vi "Update Values.vi"(0 "Portfolio en entrée":refnum<class "Portfolio.lvclass"> caption="DNL_LabVIEW Object in", 5 "With Web Update ?":bool, 11 "error in (no error)":errorcluster caption="entrée d'erreur (pas d'erreur)") -> (4 "Portfolio en sortie":refnum<class "Portfolio.lvclass"> caption="DNL_LabVIEW Object out", 6 "Tableau":string[][](array[string]), 8 "Couleurs Change (%)":u32[](array[numeric]), 10 "Couleurs Obj":u32[](array[numeric]), 12 "Couleurs Stop (%)":u32[](array[numeric]), 13 "Calc Done ?":bool, 14 "Couleurs Dividende":u32[](array[numeric]), 15 "error out":errorcluster caption="sortie d'erreur")   [LabVIEW 2012, in "Portfolio.lvclass"]
uses:
  Portfolio.lvclass
  Stocks Manager/Stock Manager Action.ctl
  Portfolio.lvclass/Portfolio.ctl
  Stock/Stock.lvclass/Stock.ctl
  Stock/Stock.lvclass
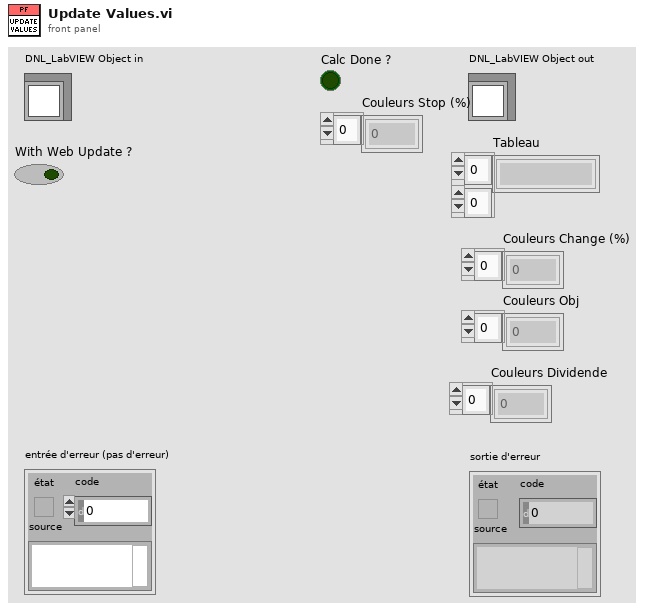
[diagram p1: front panel]
types:
  T1 = typedef "Stock Manager Action.ctl" = enum16{"Get_Stocks", "Load_Stocks", "Find_Stock_From_ISIN", "Find_Stock_From_Label", "Find_Stock_From_Symbol"}
  T2 = typedef "Stock.lvclass/Stock Parameters.ctl" = cluster{"Label":string, "Symbol":string, "Dividend":dbl, "Currency":T3, "ISIN":string, "Symbol_Suffix":string, "Last Price":dbl, "Dividend-Date":string, "Change (%)":dbl, "Objective":dbl, "Stop":dbl}
  T3 = typedef "Currencies.ctl" = enum16{"Euro", "Dollar", "Yen", "RIM", "CHF"}
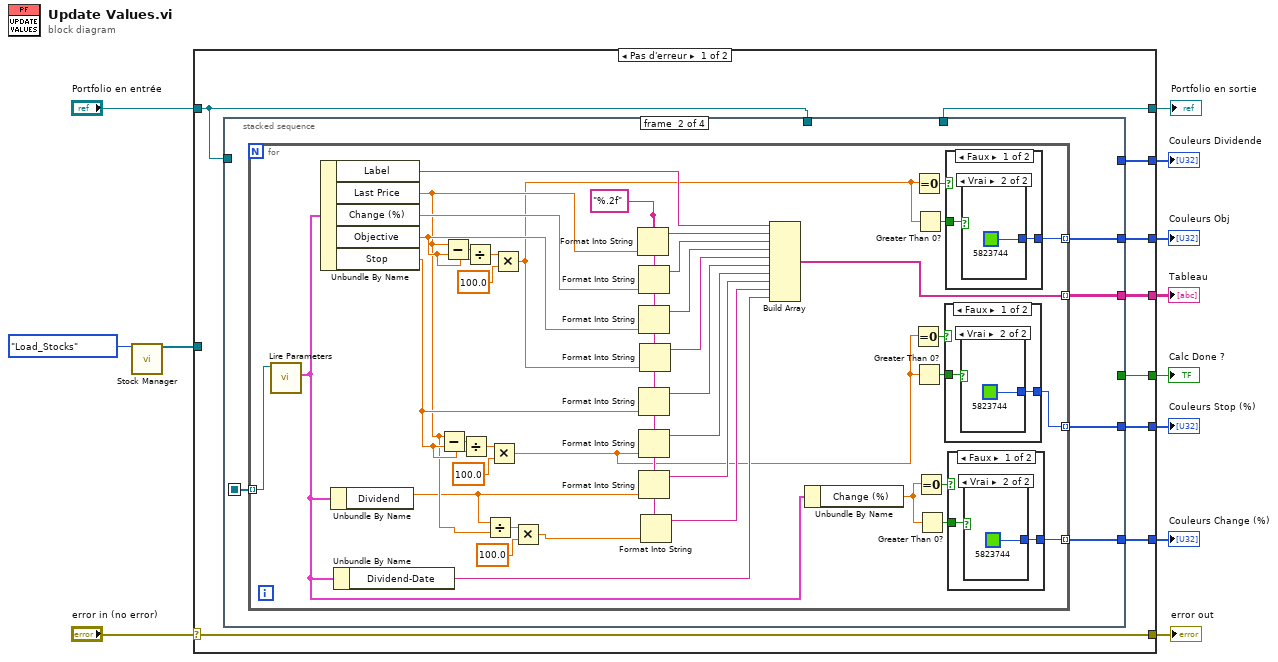
[diagram p0: block diagram]
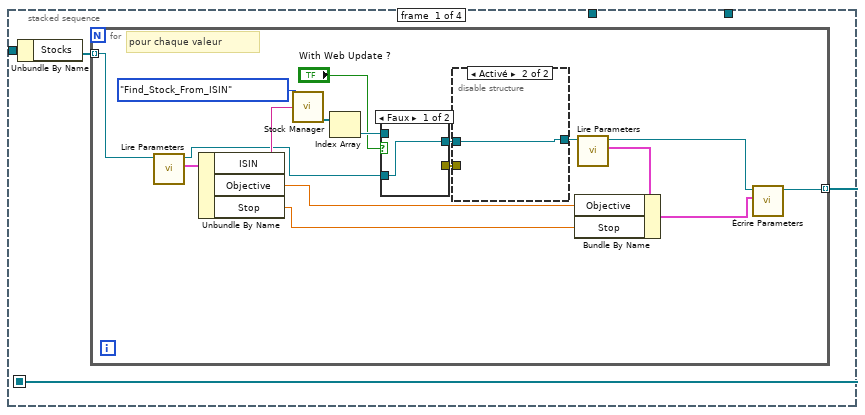
[diagram p2: hidden frame]
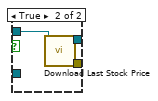
[diagram p3: hidden frame]
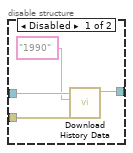
[diagram p4: hidden frame]
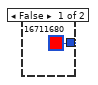
[diagram p5: hidden frame]
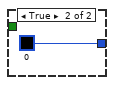
[diagram p6: hidden frame]
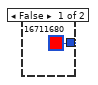
[diagram p7: hidden frame]
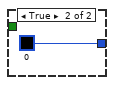
[diagram p8: hidden frame]
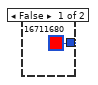
[diagram p9: hidden frame]
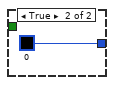
[diagram p10: hidden frame]
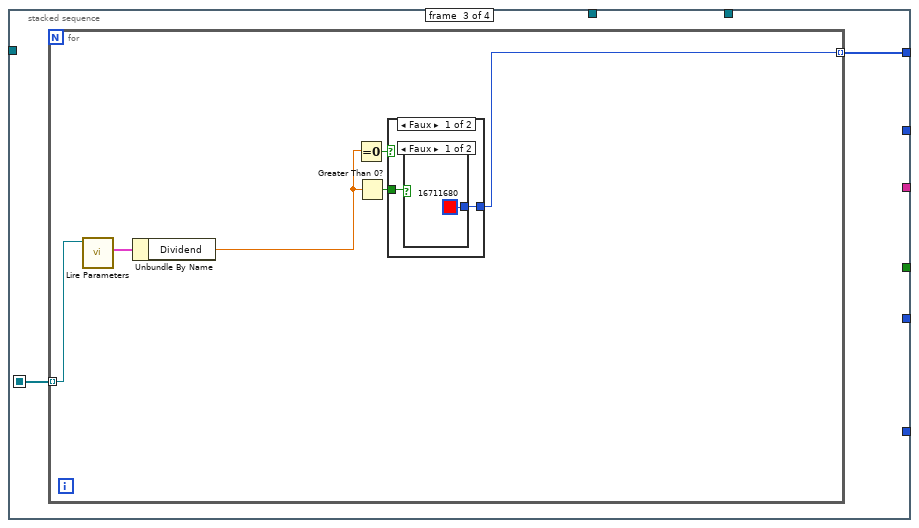
[diagram p11: hidden frame]
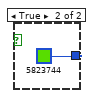
[diagram p12: hidden frame]
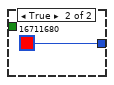
[diagram p13: hidden frame]
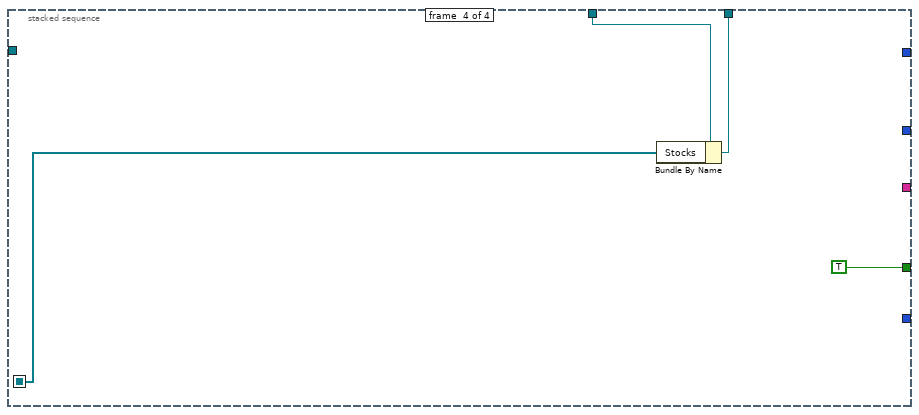
[diagram p14: hidden frame]
diagram:
  n1 = call "Stock Manager.vi"("Stock Manager Action"=Stock_Manager_Action."Load_Stocks") -> ("Stocks"=w7:refnum<class "Stock.lvclass">[])  [unwired: 12 in, 2 out]
  n2 = case shown="Pas d'erreur" "error in (no error)" {
    selector: "error in (no error)" -> [w21 w129]
    tunnel: [w21 w129] -> w12
    tunnel: [w15 w128] -> w10
    tunnel: "Portfolio en entrée" -> [w16 w128]
    tunnel: w7 -> [_ _]
    tunnel: [w20 _] -> w6
    tunnel: [w19 _] -> w5
    tunnel: [w18 _] -> w4
    tunnel: [w17 _] -> w3
    tunnel: [w14 _] -> w2
    tunnel: [w13 _] -> w1
    frame No Error {
      n3 = stacked-sequence {
        seq-local: [w22 _ _ _] -> [_ w55 w112 w125]
        tunnel: w16 -> [w24 _ _ _]
        tunnel: [_ w54 _ _] -> w20
        tunnel: [_ w53 _ _] -> w19
        tunnel: [_ w52 _ _] -> w18
        tunnel: [_ _ w111 _] -> w17
        tunnel: w16 -> [_ _ _ w127]
        tunnel: [_ _ _ w126] -> w15
        tunnel: [_ _ _ TRUE] -> w14
        tunnel: [_ w51 _ _] -> w13
        frame #0 {
          n4 = Unbundle By Name(w24) -> ("Stocks"=w23:refnum<class "Stock.lvclass">[])
          n5 = for {
            tunnel: w23 -> [w41] mode=indexing
            tunnel: [w31] -> w22 mode=indexing
            # "pour chaque valeur"
            n6 = call "Lire Parameters.vi"("Stock en entrée"=w41) -> ("Parameters"=w39:T2, "Stock en sortie"=w25:refnum<class "Stock.lvclass">)  [unwired: 9 in]
            n7 = Unbundle By Name(w39) -> ("ISIN"=w38:string, "Objective"=w28:dbl, "Stop"=w27:dbl)
            n8 = call "Stock Manager.vi"("Stock Manager Action"=Stock_Manager_Action."Find_Stock_From_ISIN", "String to find (ISIN,Label,Symbol)"=w38) -> ("Stocks Found"=w37:refnum<class "Stock.lvclass">[])  [unwired: 11 in, 2 out]
            n9 = Index Array(array=w37) -> (element=w36:refnum<class "Stock.lvclass">)  [unwired: 1 in]
            n10 = case shown="Faux" "With Web Update ?" {
              tunnel: w36 -> [_ w45]
              tunnel: [w42 w44] -> w35
              tunnel: [_ w43] -> w34
              tunnel: w25 -> [w42 _]
              frame False {
              }
              frame True {
                n11 = call "Download Last Stock Price.vi"("Share en entrée"=w45) -> ("error out"=w43:errorcluster, "Share en sortie"=w44:refnum<class "Stock.lvclass">)  [unwired: 7 in, 2 out]
              }
            }
            n12 = disable-structure shown="Activé" {
              disable-tunnel: w35 -> [w49 w50]
              disable-tunnel: w34 -> [w48 _]
              disable-tunnel: [w46 w50] -> w33
              frame Disabled {
                n13 = call "Download History Data.vi"("error in (no error)"=w48, "Min_Date"="1990", "Share en entrée"=w49) -> ("Share en sortie"=w46:refnum<class "Stock.lvclass">)  [unwired: 5 in, 3 out]
              }
              frame Enabled {
              }
            }
            n14 = call "Lire Parameters.vi"("Stock en entrée"=w33) -> ("Parameters"=w30:T2, "Stock en sortie"=w32:refnum<class "Stock.lvclass">)  [unwired: 9 in]
            n15 = Bundle By Name(cluster=w30, "Objective"=w28, "Stop"=w27) -> (w29:T2)
            n16 = call "Écrire Parameters.vi"("Parameters"=w29, "Stock en entrée"=w32) -> ("Stock en sortie"=w31:refnum<class "Stock.lvclass">)  [unwired: 9 in]
          }
        }
        frame #1 {
          n17 = for {
            tunnel: w55 -> [w95] mode=indexing
            tunnel: [w92] -> w54 mode=indexing
            tunnel: [w74] -> w53 mode=indexing
            tunnel: [w64] -> w52 mode=indexing
            tunnel: [w56] -> w51 mode=indexing
            w70 = "%.2f" ("chaîne de format")
            n18 = call "Lire Parameters.vi"("Stock en entrée"=w95) -> ("Parameters"=w68:T2)  [unwired: 9 in, 1 out]
            n19 = Unbundle By Name(w68) -> ("Label"=w93:string, "Last Price"=w71:dbl, "Change (%)"=w91:dbl, "Objective"=w87:dbl, "Stop"=w79:dbl)
            n20 = Unbundle By Name(w68) -> ("Dividend"=w60:dbl)
            n21 = Unbundle By Name(w68) -> ("Dividend-Date"=w61:string)
            n22 = Subtract(x=w71, y=w79) -> (x-y=w80:dbl)
            n23 = Subtract(x=w71, y=w87) -> (x-y=w88:dbl)
            n24 = Divide(x=w80, y=w79) -> (x/y=w81:dbl)
            n25 = Divide(x=w88, y=w87) -> (x/y=w86:dbl)
            n26 = Divide(x=w60, y=w71) -> (x/y=w73:dbl)
            n27 = Multiply(x=w81, y=100.0) -> (x*y=w57:dbl)
            n28 = Multiply(x=w86, y=100.0) -> (x*y=w65:dbl)
            n29 = Multiply(x=w73, y=100.0) -> (x*y=w69:dbl)
            n30 = Format Into String(format string=w70, w71) -> (resulting string=w94:string)  [unwired: 2 in, 1 out]
            n31 = Format Into String(format string=w70, w91) -> (resulting string=w90:string)  [unwired: 2 in, 1 out]
            n32 = Format Into String(format string=w70, w87) -> (resulting string=w89:string)  [unwired: 2 in, 1 out]
            n33 = Format Into String(format string=w70, w79) -> (resulting string=w83:string)  [unwired: 2 in, 1 out]
            n34 = Format Into String(format string=w70, w57) -> (resulting string=w78:string)  [unwired: 2 in, 1 out]
            n35 = Format Into String(format string=w70, w60) -> (resulting string=w63:string)  [unwired: 2 in, 1 out]
            n36 = Format Into String(format string=w70, w65) -> (resulting string=w84:string)  [unwired: 2 in, 1 out]
            n37 = Format Into String(format string=w70, w69) -> (resulting string=w62:string)  [unwired: 2 in, 1 out]
            n38 = Build Array(w93, w94, w90, w89, w84, w83, w78, w63, w62, w61) -> (w92:string[])
            n39 = Unbundle By Name(w68) -> ("Change (%)"=w75:dbl)
            n40 = Equal To 0?(x=w57) -> (x = 0?=w58:bool)
            n41 = Equal To 0?(x=w65) -> (x = 0?=w66:bool)
            n42 = Greater Than 0?(x=w57) -> (x > 0?=w59:bool)
            n43 = Greater Than 0?(x=w65) -> (x > 0?=w67:bool)
            n44 = Equal To 0?(x=w75) -> (x = 0?=w77:bool)
            n45 = Greater Than 0?(x=w75) -> (x > 0?=w76:bool)
            n46 = case shown="Faux" w58 {
              tunnel: [w96 u32 0 ("Color")] -> w56
              tunnel: w59 -> [w97 _]
              frame False {
                n47 = case shown="Vrai" w97 {
                  tunnel: [u32 16711680 ("Color") u32 5823744 ("Color")] -> w96
                  frame False {
                  }
                  frame True {
                  }
                }
              }
              frame True {
              }
            }
            n48 = case shown="Faux" w66 {
              tunnel: [w101 u32 0 ("Color")] -> w64
              tunnel: w67 -> [w102 _]
              frame False {
                n49 = case shown="Vrai" w102 {
                  tunnel: [u32 16711680 ("Color") u32 5823744 ("Color")] -> w101
                  frame False {
                  }
                  frame True {
                  }
                }
              }
              frame True {
              }
            }
            n50 = case shown="Faux" w77 {
              tunnel: [w106 u32 0 ("Color")] -> w74
              tunnel: w76 -> [w107 _]
              frame False {
                n51 = case shown="Vrai" w107 {
                  tunnel: [u32 16711680 ("Color") u32 5823744 ("Color")] -> w106
                  frame False {
                  }
                  frame True {
                  }
                }
              }
              frame True {
              }
            }
          }
        }
        frame #2 {
          n52 = for {
            tunnel: w112 -> [w118] mode=indexing
            tunnel: [w113] -> w111 mode=indexing
            n53 = call "Lire Parameters.vi"("Stock en entrée"=w118) -> ("Parameters"=w117:T2)  [unwired: 9 in, 1 out]
            n54 = Unbundle By Name(w117) -> ("Dividend"=w114:dbl)
            n55 = Equal To 0?(x=w114) -> (x = 0?=w116:bool)
            n56 = Greater Than 0?(x=w114) -> (x > 0?=w115:bool)
            n57 = case shown="Faux" w116 {
              tunnel: [w119 u32 16711680 ("Color")] -> w113
              tunnel: w115 -> [w120 _]
              frame False {
                n58 = case shown="Faux" w120 {
                  tunnel: [u32 16711680 ("Color") u32 5823744 ("Color")] -> w119
                  frame False {
                  }
                  frame True {
                  }
                }
              }
              frame True {
              }
            }
          }
        }
        frame #3 {
          n59 = Bundle By Name(cluster=w127, "Stocks"=w125) -> (w126:refnum<class "Portfolio.lvclass">)
        }
      }
    }
    frame Error {
    }
  }
  "error out" <- w12
  "Portfolio en sortie" <- w10
  "Tableau" <- w6
  "Couleurs Change (%)" <- w5
  "Couleurs Obj" <- w4
  "Couleurs Dividende" <- w3
  "Calc Done ?" <- w2
  "Couleurs Stop (%)" <- w1
